vi "Set Drive Output.vi"(7 "Y axis":dbl(slide) scale=0.0..10.0, 8 "X axis":dbl(slide) scale=0.0..10.0, 9 "Drive RefNum":string) -> ()   [LabVIEW 2012]
uses:
  <vilib>/Rock Robotics/WPI/RobotDrive/WPI_RobotDriveGetSetRefNum.vi
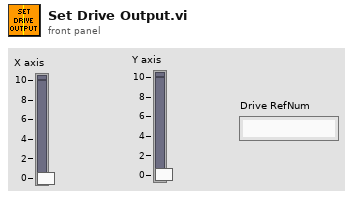
[diagram p1: front panel]
types:
  T1 = typedef "WPI_RobotDriveDevRef.ctl" = cluster{"DevStatus":errorcluster, "Motors[]":T2[], "Square Inputs":bool, "Max Output":dbl, "Isochronous":bool}
  T2 = typedef "WPI_MotorControlDeviceRef.ctl" = cluster{"DeviceStatus":errorcluster, "Type":enum16{"PWM", "CAN"}, "PWM":cluster{"Digital Module":T3, "PWM Channel":T4, "DeadBand":T5}, "CAN":cluster{"Device Number":u8, "Control Mode":T6, "Semaphore":T7, "Max Vout":dbl}, "Invert":bool, "TransformRef":T8, "InvTransformRef":T8}
  T3 = typedef "FPGA_TypedefDigitalModule.ctl" = enum16{"Digital Module 1", "Digital Module 2"}
  T4 = typedef "FPGA_DIOPWMChannel.ctl" = enum8{"PWM 1", "PWM 2", "PWM 3", "PWM 4", "PWM 5", "PWM 6", "PWM 7", "PWM 8", "PWM 9", "PWM 10", "Invalid"}
  T5 = typedef "WPI_PWMDeadband.ctl" = cluster{"Name":string, "maxPositivePwm":i32, "minPositivePwm":i32, "centerPwm":i32, "maxNegativePwm":i32, "minNegativePwm":i32, "angularRange":u16}
  T6 = typedef "WPI_CANJaguar_ControlMode.ctl" = enum8{"Percent VBus", "Current", "Speed", "Position", "Voltage"}
  T7 = typedef "Semaphore RefNum" = refnum<k1>
  T8 = typedef "WPI_PWMTransform_ConPane.ctl" = refnum<vi>
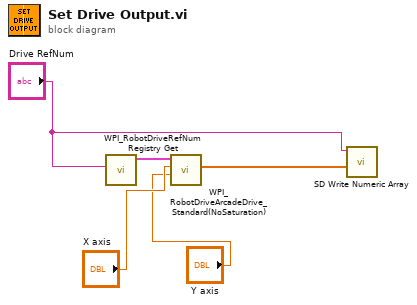
[diagram p0: block diagram]
diagram:
  n1 = call <vilib>:"WPI_RobotDriveRefNum Registry Get.vi"("refnum name"="Drive RefNum") -> ("RobotDriveDevRef"=w4:T1)  [unwired: 1 in, 9 out]
  n2 = call <vilib>:"WPI_RobotDriveArcadeDrive_Standard(NoSaturation).vi"("Y axis value"="Y axis", "X axis value"="X axis", "RobotDriveDevRef"=w4) -> ("Motor Values"=w5:dbl[])  [unwired: 1 in, 7 out]
  n3 = call <vilib>:"SD Write Numeric Array.vi"("Numeric Array"=w5, "Name"="Drive RefNum") -> ()  [unwired: 8 in, 2 out]
